vi "ResampleXY.vi"(7 "Interpolation Distance":dbl format="%#_13g", 8 "error in (no error)":errorcluster, 9 "t":dbl[](array[numeric]), 10 "Y":dbl[](array[numeric]), 11 "X":dbl[](array[numeric])) -> (0 "error out":errorcluster, 2 "Resampled Y":dbl[](array[numeric]), 3 "Resampled X":dbl[](array[numeric]))   [LabVIEW 2019, in "Tool Object.lvclass"]
uses:
  Tool Object.lvclass
  <vilib>/Analysis/1siggen.llb/Ramp Pattern by Samples.vi
  <vilib>/gmath/NI_Gmath.lvlib
  <vilib>/Analysis/NI_AALBase.lvlib
  Tool Path/Tool Path.lvclass
panel:
  out "XY Graph":cluster{"X":dbl[], "Y":dbl[]}(graph)
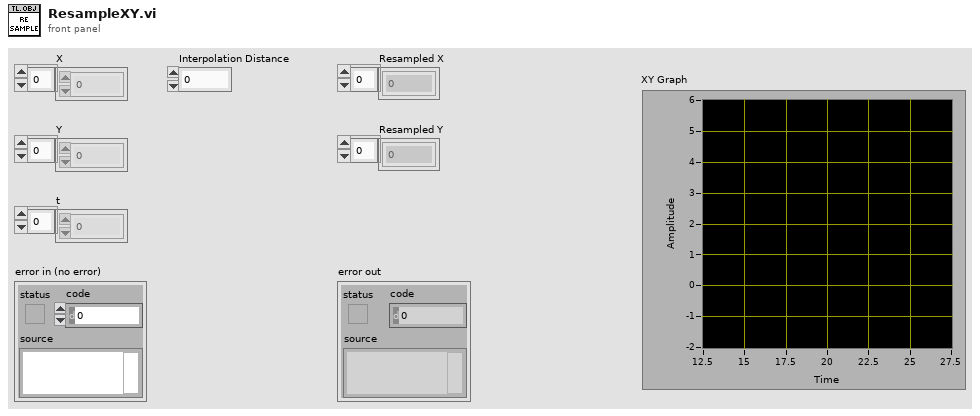
[diagram p1: front panel]
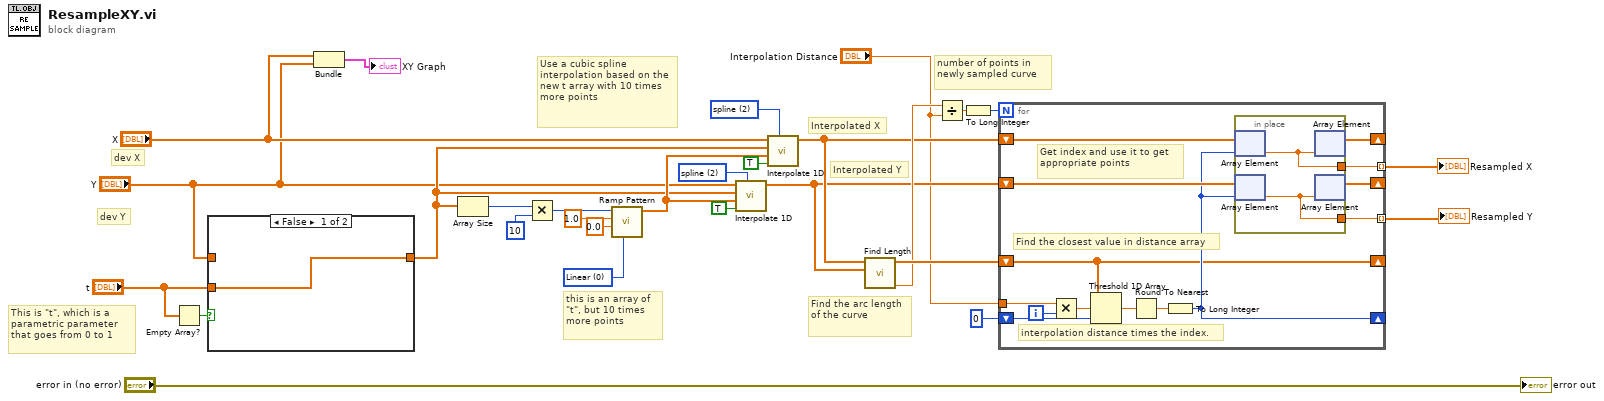
[diagram p0: block diagram]
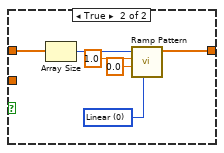
[diagram p2: hidden frame]
diagram:
  w24 = u16 0 items=["Linear", "Logarithmic"] ("type")
  w25 = 2 items=["nearest", "linear", "spline", "cubic Hermite", "Lagrange"] ("method")
  w26 = 2 items=["nearest", "linear", "spline", "cubic Hermite", "Lagrange"] ("method")
  # "number of points in newly sampled curve"
  # "Find the arc length of the curve"
  # "Use a cubic spline interpolation based on the new t array with 10 times more points"
  # "this is an array of \"t\", but 10 times more points"
  # "dev X"
  # "dev Y"
  # "This is \"t\", which is a parametric parameter that goes from 0 to 1"
  # "Interpolated Y"
  # "Interpolated X"
  n1 = Empty Array?(array="t") -> (empty?=w7:bool)
  n2 = case shown="False" w7 {
    tunnel: "t" -> [w29 _]
    tunnel: [w29 w31] -> w5
    tunnel: "Y" -> [_ w30]
    frame False {
    }
    frame True {
      w35 = u16 0 items=["Linear", "Logarithmic"] ("type")
      n3 = Array Size(array=w30) -> (size(s)=w32:i32)
      n4 = call-poly <vilib>:"Ramp Pattern.vi"("type"=w35, "start"=0.0, "end"=1.0, "samples"=w32) -> ("Ramp Pattern"=w31:dbl[])  [unwired: 6 in, 1 out]
    }
  }
  n5 = Bundle("X"="X", "Y"="Y") -> (→"XY Graph":cluster{"X":dbl[], "Y":dbl[]})  [unwired: 1 in]
  n6 = Array Size(array=w5) -> (size(s)=w14:i32)
  n7 = Multiply(x=w14, y=10 ("x")) -> (x*y=w20:i32)
  n8 = call-poly <vilib>:"Ramp Pattern.vi"("type"=w24, "start"=0.0, "end"=1.0, "samples"=w20) -> ("Ramp Pattern"=w19:dbl[])  [unwired: 6 in, 1 out]
  n9 = call <vilib>:"Interpolate 1D.vi"("method"=w26, "X is monotonic"=TRUE, "xi"=w19, "X"=w5, "Y"="Y") -> ("yi"=w17:dbl[])  [unwired: 4 in, 2 out]
  n10 = call <vilib>:"Interpolate 1D.vi"("method"=w25, "X is monotonic"=TRUE, "xi"=w19, "X"=w5, "Y"="X") -> ("yi"=w18:dbl[])  [unwired: 4 in, 2 out]
  n11 = call "Find Length.vi"("Y"=w17, "X"=w18) -> ("Total Length"=w21:dbl, "Cumulative Length"=w22:dbl[])  [unwired: 6 in, 2 out]
  n12 = Divide(x=w21, y="Interpolation Distance") -> (x/y=w12:dbl)
  n13 = To Long Integer(number=w12) -> (32bit integer=w11:i32)
  n14 = for {
    N: w11 -> [_]
    tunnel: "Interpolation Distance" -> [w49]
    shift-right: [w44] -> _
    shift-left: w18 -> [w46]
    shift-right: [w43] -> _
    shift-left: w17 -> [w45]
    tunnel: [w42] -> w9 mode=indexing
    tunnel: [w41] -> w10 mode=indexing
    shift-right: [w36] -> _
    shift-left: w22 -> [w36]
    shift-right: [w39] -> _
    shift-left: 0 -> [w40]
    i -> [w48]
    # "interpolation distance times the index."
    # "Get index and use it to get appropriate points"
    # "Find the closest value in distance array"
    n15 = Multiply(x=w49, y=w48) -> (x*y=w47:dbl)
    n16 = Threshold 1D Array(1:w40, 2:w47, 3:w36) -> (0:w38:dbl)
    n17 = Round To Nearest(number=w38) -> (nearest integer value=w37:dbl)
    n18 = To Long Integer(number=w37) -> (32bit integer=w39:i32)
    n19 = in-place {
      in-place-border: [w51] -> w41
      in-place-border: [w50] -> w42
      n20 = in-place-array #1(w46, w39) -> (w51:dbl)
      n21 = in-place-array #2(w45, w39) -> (w50:dbl)
      n22 = in-place-array #1(w51) -> (w44:dbl[])  [unwired: 1 out]
      n23 = in-place-array #2(w50) -> (w43:dbl[])  [unwired: 1 out]
    }
  }
  "Resampled Y" <- w9
  "Resampled X" <- w10
  "error out" <- "error in (no error)"
